vi "Create New Assert.vi"(6 "Variant in":variant, 7 "Shift Pressed?":bool, 8 "error in (no error)":errorcluster, 10 "QD Combo Box Ref":refnum<vi>, 11 "QD Launch VI Ref":refnum<vi>) -> (0 "error out":errorcluster, 4 "Variant out":variant)   [LabVIEW 2016]
doc: "Allows the user to define and insert a new assert statement onto a wire - supports I32, Double, String and Boolean data types currently\n\nDefault Shortcut - S"
panel:
  in  "Undo Name":string="Quick Drop Keyboard Shortcut"
  # "Do not change the connector pane of this VI.\n\nSee the block diagram for directions on how to use this template."
  # "Specify the name of the Undo transaction"
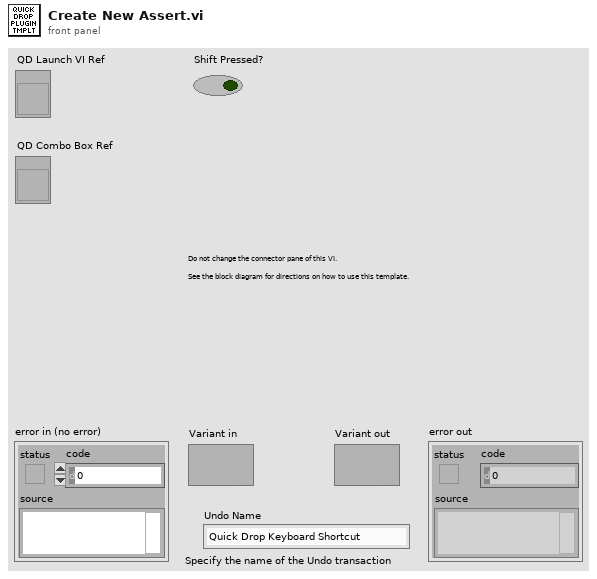
[diagram p1: front panel]
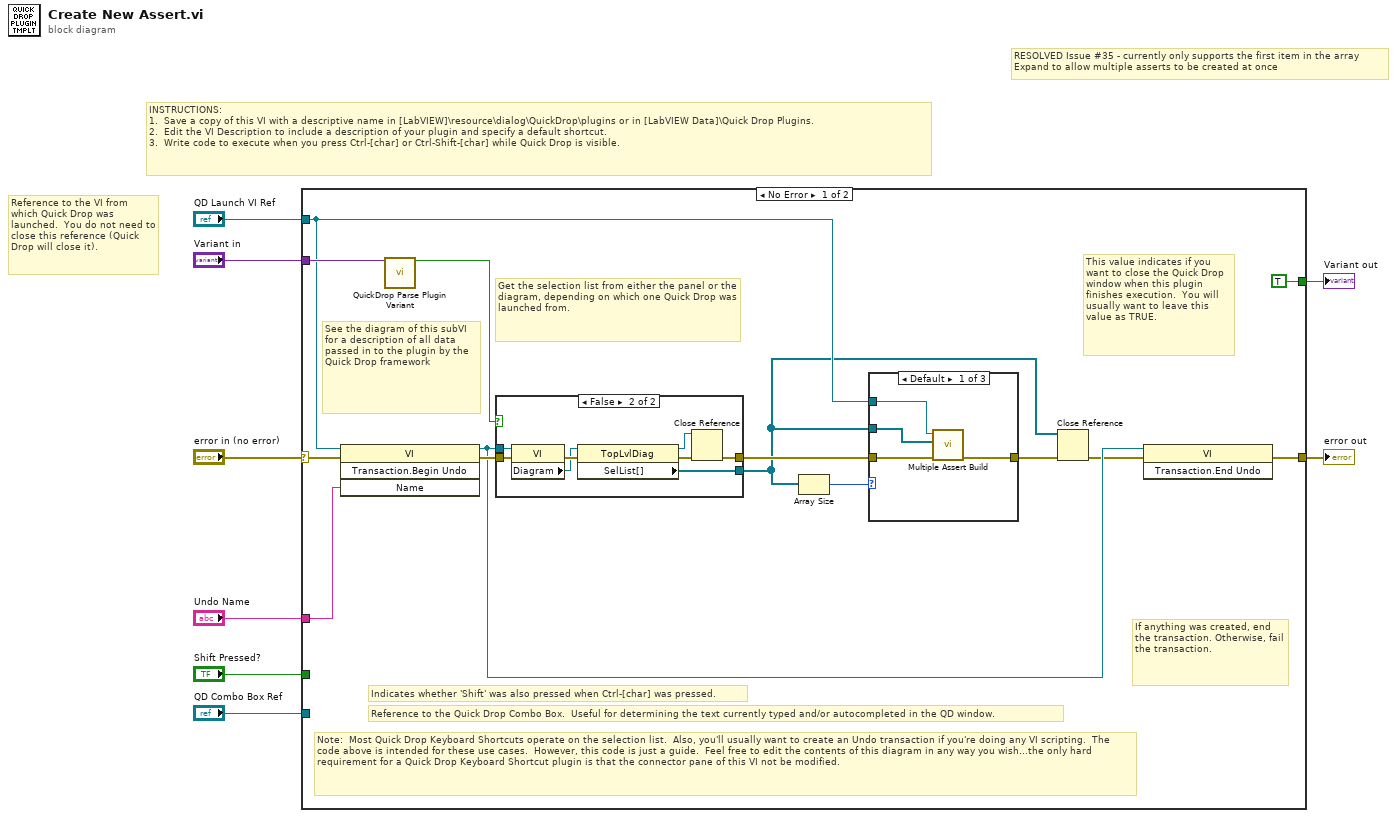
[diagram p0: block diagram]
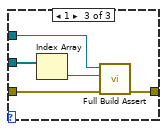
[diagram p3: hidden frame]
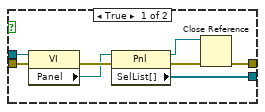
[diagram p4: hidden frame]
diagram:
  # "RESOLVED Issue #35 - currently only supports the first item in the array\nExpand to allow multiple asserts to be created at once"
  # "Reference to the VI from which Quick Drop was launched.  You do not need to close this reference (Quick Drop will close it)."
  # "INSTRUCTIONS:\n1.  Save a copy of this VI with a descriptive name in [LabVIEW]\\resource\\dialog\\QuickDrop\\plugins or in [LabVIEW Data]\\Quick Drop Plugins.\n2.  Edit the VI Description to include a description of your plugin and specify a default shortcut. \n3.  Write code to execute when you press Ctrl-[char] or Ctrl-Shift-[char] while Quick Drop is visible."
  n1 = case shown="No Error" "error in (no error)" {
    selector: "error in (no error)" -> [w21 w49]
    tunnel: [w16 w49] -> w7
    tunnel: "QD Launch VI Ref" -> [w11 _]
    tunnel: "Shift Pressed?" -> [_ _]
    tunnel: "QD Combo Box Ref" -> [_ _]
    tunnel: "Variant in" -> [w22 _]
    tunnel: "Undo Name" -> [w20 _]
    tunnel: [TRUE _] -> w1
    frame No Error {
      # "Note:  Most Quick Drop Keyboard Shortcuts operate on the selection list.  Also, you'll usually want to create an Undo transaction if you're doing any VI scripting.  The code above is intended for these use cases.  However, this code is just a guide.  Feel free to edit the contents of this diagram in any way you wish...the only hard requirement for a Quick Drop Keyboard Shortcut plugin is that the connector pane of this VI not be modified."
      # "Get the selection list from either the panel or the diagram, depending on which one Quick Drop was launched from."
      # "If anything was created, end the transaction. Otherwise, fail the transaction."
      # "This value indicates if you want to close the Quick Drop window when this plugin finishes execution.  You will usually want to leave this value as TRUE."
      # "See the diagram of this subVI for a description of all data passed in to the plugin by the Quick Drop framework"
      # "Reference to the Quick Drop Combo Box.  Useful for determining the text currently typed and/or autocompleted in the QD window."
      # "Indicates whether 'Shift' was also pressed when Ctrl-[char] was pressed."
      n2 = invoke class="VI" method="Transaction.Begin Undo"(reference=w11, error in=w21, "Name"=w20) -> (reference out=w15:refnum<vi>, error out=w17:errorcluster)  [unwired: 1 in, 2 out]
      n3 = call <vilib>:"QuickDrop Parse Plugin Variant.vi"("QDKS Variant in"=w22) -> ("QD Launch VI Panel?"=w18:bool)  [unwired: 12 in, 2 out]
      n4 = case shown="False" w18 {
        tunnel: w17 -> [w40 w48]
        tunnel: w15 -> [w39 w47]
        tunnel: [w34 w42] -> w13
        tunnel: [w33 w41] -> w9
        frame True {
          n5 = property class="VI"(reference=w39, error in=w40) -> (error out=w38:errorcluster, "Panel"=w37:refnum<vi>)  [unwired: 1 out]
          n6 = property class="Pnl"(reference=w37, error in=w38) -> (reference out=w35:refnum<vi>, error out=w36:errorcluster, "SelList[]"=w33:refnum<vi>[])
          n7 = Close Reference(reference=w35, error in (no error)=w36) -> (error out=w34:errorcluster)
        }
        frame False {
          n8 = property class="VI"(reference=w47, error in=w48) -> (error out=w46:errorcluster, "Diagram"=w45:refnum<vi>)  [unwired: 1 out]
          n9 = property class="TopLvlDiag"(reference=w45, error in=w46) -> (reference out=w43:refnum<vi>, error out=w44:errorcluster, "SelList[]"=w41:refnum<vi>[])
          n10 = Close Reference(reference=w43, error in (no error)=w44) -> (error out=w42:errorcluster)
        }
      }
      n11 = Array Size(array=w9) -> (size(s)=w10:i32)
      n12 = case shown="Default" w10 {
        tunnel: w13 -> [w24 w27 w32]
        tunnel: [w23 w27 w31] -> w12
        tunnel: w11 -> [w25 _ w30]
        tunnel: w9 -> [w26 _ w28]
        frame Default {
          n13 = call "Multiple Assert Build.vi"("error in (no error)"=w24, "GObj Array"=w26, "VI in"=w25) -> ("error out"=w23:errorcluster)  [unwired: 8 in]
        }
        frame 0 {
        }
        frame 1 {
          n14 = Index Array(array=w28) -> (element=w29:refnum<vi>)  [unwired: 1 in]
          n15 = call "Full Build Assert.vi"("error in (no error)"=w32, "GObj Refnum"=w29, "VI in"=w30) -> ("error out"=w31:errorcluster)  [unwired: 8 in]
        }
      }
      n16 = Close Reference(reference=w9, error in (no error)=w12) -> (error out=w14:errorcluster)
      n17 = invoke class="VI" method="Transaction.End Undo"(reference=w15, error in=w14) -> (error out=w16:errorcluster)  [unwired: 1 in, 2 out]
    }
    frame Error {
    }
  }
  "error out" <- w7
  "Variant out" <- w1
